vi "Run Step.vi"(8 "error in (no error)":errorcluster, 9 "result allocation":T1, 10 "parameters":T1, 11 "String Compare in":refnum<class "String Compare.lvclass">) -> (0 "error out":errorcluster, 1 "results":T1, 2 "parameter allocation":T1, 3 "String Compare out":refnum<class "String Compare.lvclass">)   [LabVIEW 2015, in "String Compare.lvclass"]
uses:
  String Compare.lvclass
  <vilib>/NI/Tag Bus/table/data table.ctl
  String Compare.lvclass/String Compare.ctl
  <vilib>/NI/Tag Bus/table/data polymorphs/read one/read String.vi
  <vilib>/NI/Tag Bus/table/data polymorphs/write one/write Boolean.vi
  <vilib>/regexp/Match Regular Expression.xnode
  <vilib>/NI/Tag Bus/table/data table.lvlib
panel:
  out "Pass/Fail?":bool
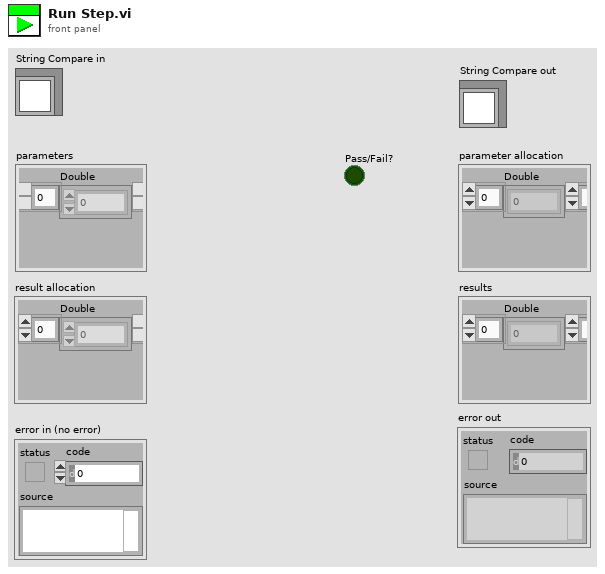
[diagram p1: front panel]
types:
  T1 = typedef "tag bus.lvlib/data table.lvlib/data table.ctl" = cluster{"Double":dbl[], "Single":sgl[], "I64":i64[], "I32":i32[], "I16":i16[], "I8":i8[], "U64":u64[], "U32":u32[], "U16":u16[], "U8":u8[], "Boolean":bool[], "String":string[], "Array of Double":cluster{"DBL Array":dbl[]}[], "Array of Single":cluster{"SGL Array":sgl[]}[], "Array of I64":cluster{"I64 Array":i64[]}[], "Array of I32":cluster{"I32 Array":i32[]}[], "Array of I16":cluster{"I16 Array":i16[]}[], "Array of I8":cluster{"I8 Array":i8[]}[], "Array of U64":cluster{"U64 Array":u64[]}[], "Array of U32":cluster{"U32 Array":u32[]}[], "Array of U16":cluster{"U16 Array":u16[]}[], "Array of U8":cluster{"U8 Array":u8[]}[], "Array of Boolean":cluster{"Boolean Array":bool[]}[], "Array of String":cluster{"String Array":string[]}[]}
  T2 = typedef "Mode.ctl" = enum16{"Compare Strings", "Match Regex"}
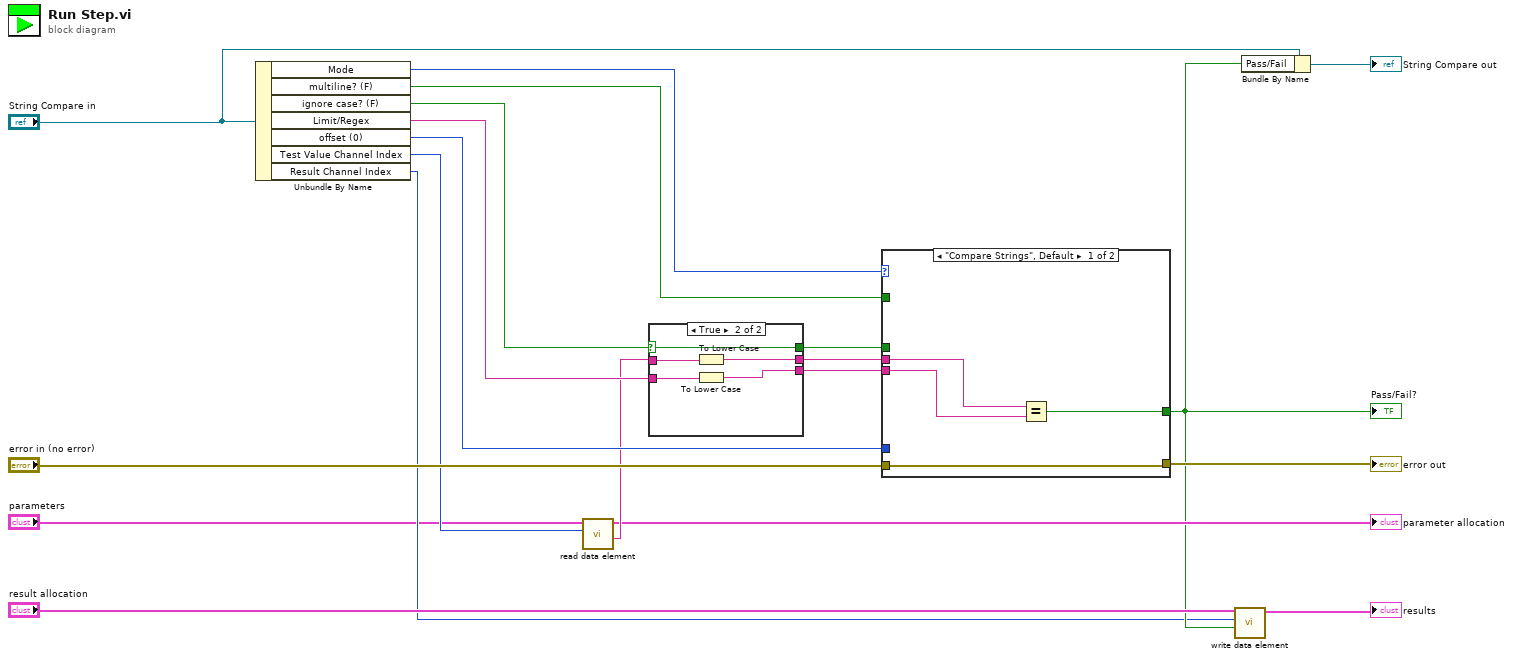
[diagram p0: block diagram]
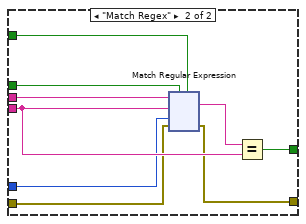
[diagram p3: hidden frame]
diagram:
  n1 = Unbundle By Name("String Compare in") -> ("Mode"=w17:T2, "multiline? (F)"=w13:bool, "ignore case? (F)"=w14:bool, "Limit/Regex"=w16:string, "offset (0)"=w15:i32, "Test Value Channel Index"=w10:i32, "Result Channel Index"=w2:i32)
  n2 = call-poly <vilib>:"read data element.vi"("index"=w10, "data table in"="parameters") -> ("value"=w9:string, "data table out"=→"parameter allocation":T1)  [unwired: 8 in]
  n3 = case shown="True" w14 {
    selector: w14 -> [w23 w24]
    tunnel: w9 -> [w22 w28]
    tunnel: w16 -> [w21 w26]
    tunnel: [w22 w27] -> w20
    tunnel: [w21 w25] -> w19
    tunnel: [w23 w24] -> w18
    frame False {
    }
    frame True {
      n4 = To Lower Case(string=w28) -> (all lower case string=w27:string)
      n5 = To Lower Case(string=w26) -> (all lower case string=w25:string)
    }
  }
  n6 = case shown="\"Compare Strings\", Default" w17 {
    tunnel: w20 -> [w32 w41]
    tunnel: w19 -> [w31 w39]
    tunnel: [w30 w38] -> w3
    tunnel: w18 -> [_ w37]
    tunnel: w13 -> [_ w36]
    tunnel: w15 -> [_ w35]
    tunnel: "error in (no error)" -> [w29 w34]
    tunnel: [w29 w33] -> w11
    frame "Compare Strings", Default {
      n7 = Equal?(x=w32, y=w31) -> (x = y?=w30:bool)
    }
    frame "Match Regex" {
      n8 = xnode "Match Regular Expression"("input string"=w41, "regular expression"=w39, "offset (0)"=w35, "error in"=w34, "ignore case? (F)"=w37, "multiline? (F)"=w36) -> ("whole match"=w40:string, "error out"=w33:errorcluster)  [unwired: 3 out]
      n9 = Equal?(x=w40, y=w39) -> (x = y?=w38:bool)
    }
  }
  "error out" <- w11
  "Pass/Fail?" <- w3
  n10 = call-poly <vilib>:"write data element.vi"("value"=w3, "index"=w2, "data table in"="result allocation") -> ("data table out"=→"results":T1)  [unwired: 8 in]
  n11 = Bundle By Name(cluster="String Compare in", "Pass/Fail"=w3) -> (→"String Compare out":refnum<class "String Compare.lvclass">)
